vi "Time(string_number).vi"() -> ()   [LabVIEW 2012]
panel:
  in  "Datetime string array":string[](array[string])
  out "Time stamp array":timestamp[](array[timestamp])
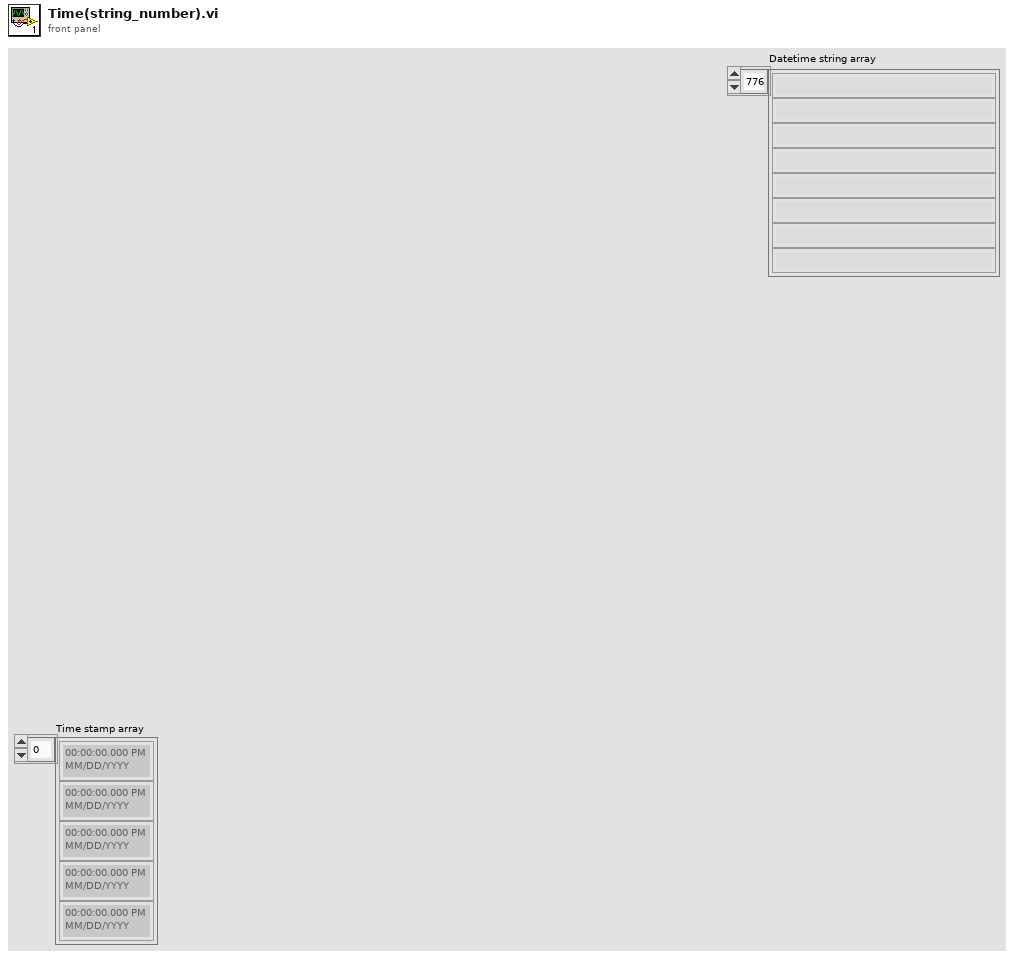
[diagram p1: front panel]
types:
  T1 = typedef "LVDateTimeRec.ctl" = cluster{"fractional second":dbl, "second":i32, "minute":i32, "hour":i32, "day of month":i32, "month":i32, "year":i32, "day of week":i32, "day of year":i32, "DST":i32}
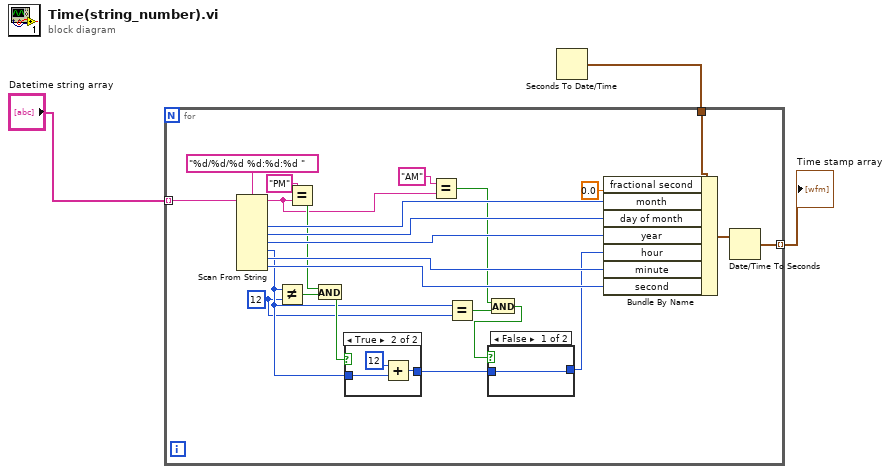
[diagram p0: block diagram]
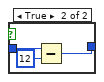
[diagram p2: hidden frame]
diagram:
  n1 = Seconds To Date/Time() -> (date time rec=w3:T1)  [unwired: 2 out]
  n2 = for {
    tunnel: "Datetime string array" -> [w27] mode=indexing
    tunnel: w3 -> [w25]
    tunnel: [w23] -> w2 mode=indexing
    w5 = 12 ("y")
    n3 = Scan From String(format string="%d/%d/%d %d:%d:%d ", input string=w27) -> (remaining string=w12:string, output 1=w19:i32, output 2=w18:i32, output 3=w17:i32, output 4=w6:i32, output 5=w21:i32, output 6=w20:i32)  [unwired: 2 in, 8 out]
    n4 = Not Equal?(x=w6, y=w5) -> (x != y?=w10:bool)
    n5 = Equal?(x="PM", y=w12) -> (x = y?=w15:bool)
    n6 = And(x=w15, y=w10) -> (x .and. y?=w14:bool)
    n7 = case shown="True" w14 {
      tunnel: w6 -> [w32 w34]
      tunnel: [w32 w35] -> w9
      frame False {
      }
      frame True {
        n8 = Add(x=12, y=w34) -> (x+y=w35:i32)
      }
    }
    n9 = Equal?(x="AM", y=w12) -> (x = y?=w11:bool)
    n10 = Equal?(x=w6, y=w5) -> (x = y?=w7:bool)
    n11 = And(x=w11, y=w7) -> (x .and. y?=w4:bool)
    n12 = case shown="False" w4 {
      tunnel: w9 -> [w28 w31]
      tunnel: [w28 w30] -> w8
      frame False {
      }
      frame True {
        n13 = Subtract(x=w31, y=12) -> (x-y=w30:i32)
      }
    }
    n14 = Bundle By Name(cluster=w25, "fractional second"=0.0, "month"=w19, "day of month"=w18, "year"=w17, "hour"=w8, "minute"=w21, "second"=w20) -> (w24:T1)
    n15 = Date/Time To Seconds(2:w24) -> (0:w23:timestamp)  [unwired: 1 out]
  }
  "Time stamp array" <- w2
